vi "PrintDlgEx.vi"(6 "error in (no error)":errorcluster) -> (0 "error out":errorcluster, 1 "Port":string, 2 "Printer":string, 3 "Driver":string, 4 "Cancelled?":bool)   [LabVIEW 2011]
uses:
  comdlg32.dll
panel:
  out "HRESULT":u32 format="%.0x"
  # "x80070057 = Invalid argument"
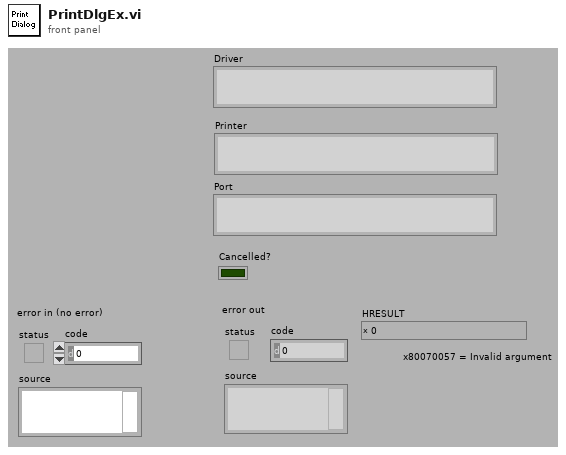
[diagram p1: front panel]
types:
  T1 = cluster{"lStructSize":i32, "hwndOwner":u32, "hDevMode":i32, "hDevNames":i32, "hDC":i32, "Flags":i32, "Flags2":i32, "ExclusionFlags":i32, "nPageRanges":i32, "nMaxPageRanges":i32, "lpPageRanges":i32, "nMinPage":i32, "nMaxPage":i32, "nCopies":i32, "hInstance":i32, "lpPrintTemplateName":i32, "lpCallback":i32, "nPropertyPages":i32, "*lphPropertyPages":i32, "nStartPage":i32, "dwResultAction":i32}
  T2 = typedef "hWnd.ctl" = refnum<k1>
  T3 = cluster{"wDriverOffset":u16, "wDeviceOffset":u16, "wOutputOffset":u16, "wDefault":u16}
  T4 = cluster{"wDriverOffset":i32, "wDeviceOffset":i32, "wOutputOffset":i32, "wDefault":i32}
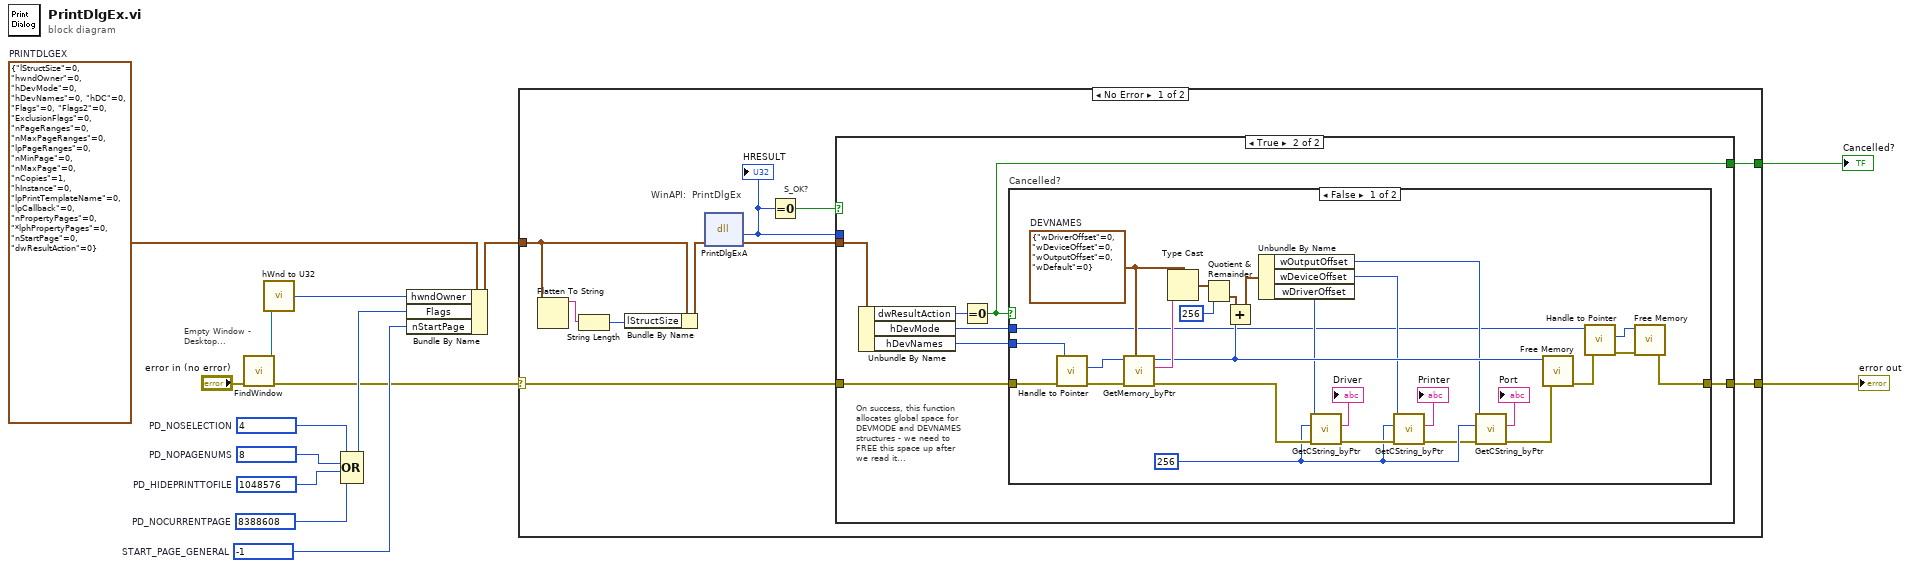
[diagram p0: block diagram]
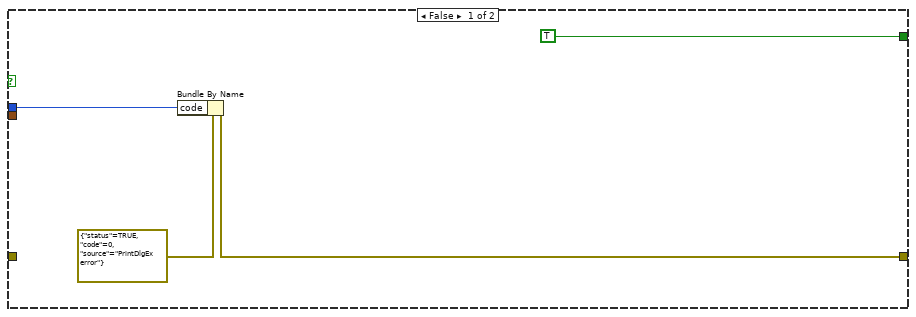
[diagram p2: hidden frame]
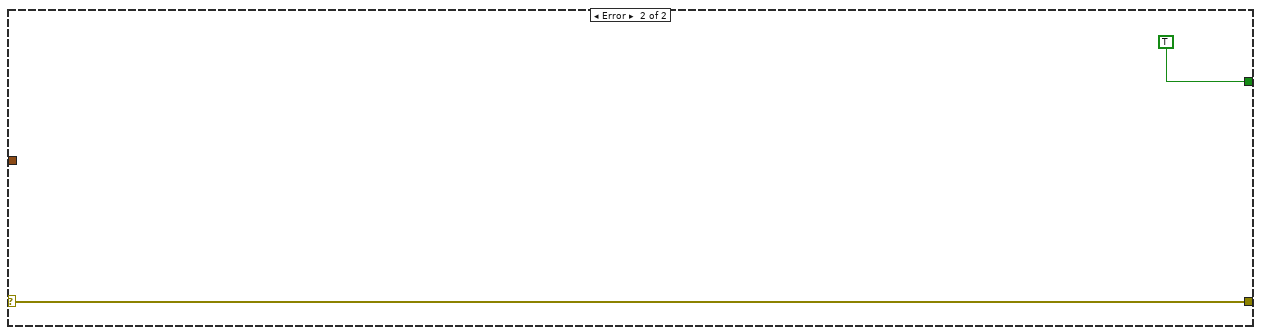
[diagram p4: hidden frame]
diagram:
  w3 = -1  # START_PAGE_GENERAL
  w4 = 4  # PD_NOSELECTION
  w5 = 8388608  # PD_NOCURRENTPAGE
  w7 = 1048576  # PD_HIDEPRINTTOFILE
  w8 = 8  # PD_NOPAGENUMS
  w12 = T1 {"lStructSize"=0, "hwndOwner"=0, "hDevMode"=0, "hDevNames"=0, "hDC"=0, "Flags"=0, "Flags2"=0, "ExclusionFlags"=0, "nPageRanges"=0, "nMaxPageRanges"=0, "lpPageRanges"=0, "nMinPage"=0, "nMaxPage"=0, "nCopies"=1, "hInstance"=0, "lpPrintTemplateName"=0, "lpCallback"=0, "nPropertyPages"=0, "*lphPropertyPages"=0, "nStartPage"=0, "dwResultAction"=0}  # PRINTDLGEX
  # "Empty Window -\nDesktop..."
  n1 = call "FindWindow.vi"("error in (no error)"="error in (no error)") -> ("error out"=w2:errorcluster, "hWnd"=w10:T2)  [unwired: 1 in, 6 out]
  n2 = call "hWnd to U32.vi"("hWnd"=w10) -> ("hWnd"=w9:u32)  [unwired: 4 out]
  n3 = Compound Arithmetic op=OR(w4, w8, w7, w5) -> (w6:i32)
  n4 = Bundle By Name(cluster=w12, "hwndOwner"=w9, "Flags"=w6, "nStartPage"=w3) -> (w11:T1)
  n5 = case shown="No Error" w2 {
    selector: w2 -> [w20 w65]
    tunnel: [w24 w65] -> w13
    tunnel: w11 -> [w16 _]
    tunnel: [w19 TRUE] -> w1
    frame No Error {
      # "WinAPI:  PrintDlgEx"
      # "S_OK?"
      n6 = Flatten To String(anything=w16) -> (data string=w18:string)  [unwired: 1 in, 4 out]
      n7 = String Length(string=w18) -> (length=w17:i32)
      n8 = Bundle By Name(cluster=w16, "lStructSize"=w17) -> (w15:T1)
      n9 = dll-call lib="comdlg32.dll" fn="PrintDlgExA"("PRINTDLGEX"=w15) -> ("HRESULT"=w21:u32, "PRINTDLGEX"=w23:T1)  [unwired: 3 in, 2 out]
      "HRESULT" <- w21
      n10 = Equal To 0?(x=w21) -> (x = 0?=w22:bool)
      n11 = case shown="True" w22 {
        tunnel: w23 -> [_ w35]
        tunnel: w20 -> [_ w34]
        tunnel: [w26 w32] -> w24
        tunnel: w21 -> [w28 _]
        tunnel: [TRUE w30] -> w19
        frame False {
          n12 = Bundle By Name(cluster=errorcluster {"status"=TRUE, "code"=0, "source"="PrintDlgEx error"} ("error out"), "code"=w28) -> (w26:errorcluster)
        }
        frame True {
          # "On success, this function\nallocates global space for \nDEVMODE and DEVNAMES\nstructures - we need to\nFREE this space up after\nwe read it..."
          n13 = Unbundle By Name(w35) -> ("dwResultAction"=w31:i32, "hDevMode"=w29:i32, "hDevNames"=w33:i32)
          n14 = Equal To 0?(x=w31) -> (x = 0?=w30:bool)
          n15 = case "Cancelled?" shown="False" w30 {
            tunnel: w34 -> [w41 w63]
            tunnel: w33 -> [w62 _]
            tunnel: [w36 w63] -> w32
            tunnel: w29 -> [w40 _]
            frame False {
              w46 = 256 ("MaxSize")
              w59 = T3 {"wDriverOffset"=0, "wDeviceOffset"=0, "wOutputOffset"=0, "wDefault"=0}  # DEVNAMES
              n16 = call "Handle to Pointer.vi"("error in (no error)"=w41, "Handle"=w62) -> ("error out"=w61:errorcluster, "Pointer"=w58:i32)  [unwired: 4 out]
              n17 = call "GetMemory_byPtr.vi"("Data Type"=w59, "error in (no error)"=w61, "Pointer"=w58) -> ("error out"=w56:errorcluster, "data"=w60:string, "Duplicate Pointer"=w52:i32)  [unwired: 1 in, 2 out]
              n18 = Type Cast(type=w59, x=w60) -> (*(type *) &x=w55:T3)
              n19 = Quotient & Remainder(x=w55, y=u16 256) -> (floor(x/y)=w53:T3)  [unwired: 1 out]
              n20 = Add(x=w53, y=w52) -> (x+y=w51:T4)
              n21 = Unbundle By Name(w51) -> ("wOutputOffset"=w42:i32, "wDeviceOffset"=w48:i32, "wDriverOffset"=w50:i32)
              n22 = call "GetCString_byPtr.vi"("error in (no error)"=w56, "MaxSize"=w46, "C String Pointer"=w50) -> ("error out"=w54:errorcluster, "String"=→"Driver":string)  [unwired: 4 out]
              n23 = call "GetCString_byPtr.vi"("error in (no error)"=w54, "MaxSize"=w46, "C String Pointer"=w48) -> ("error out"=w45:errorcluster, "String"=→"Printer":string)  [unwired: 4 out]
              n24 = call "GetCString_byPtr.vi"("error in (no error)"=w45, "MaxSize"=w46, "C String Pointer"=w42) -> ("error out"=w44:errorcluster, "String"=→"Port":string)  [unwired: 4 out]
              n25 = call "Free Memory.vi"("error in (no error)"=w44, "Pointer"=w52) -> ("error out"=w39:errorcluster)  [unwired: 5 out]
              n26 = call "Handle to Pointer.vi"("error in (no error)"=w39, "Handle"=w40) -> ("error out"=w38:errorcluster, "Pointer"=w37:i32)  [unwired: 4 out]
              n27 = call "Free Memory.vi"("error in (no error)"=w38, "Pointer"=w37) -> ("error out"=w36:errorcluster)  [unwired: 5 out]
            }
            frame True {
            }
          }
        }
      }
    }
    frame Error {
    }
  }
  "error out" <- w13
  "Cancelled?" <- w1
